vi "initialiseFields.vi"(8 "error in (no error)":errorcluster, 11 "ScanCreator in":refnum<class "ScanCreator.lvclass">) -> (0 "error out":errorcluster, 3 "ScanCreator out":refnum<class "ScanCreator.lvclass">)   [LabVIEW 2011, in "Views.lvlib" / "ScriptEditor.lvlib" / "ScanCreator.lvclass"]
uses:
  ScanCreator.lvclass
  ScanCreator.lvclass/ScanCreator.ctl
  Tools/Scripting/ScriptingEvent/ScriptEvent.lvclass
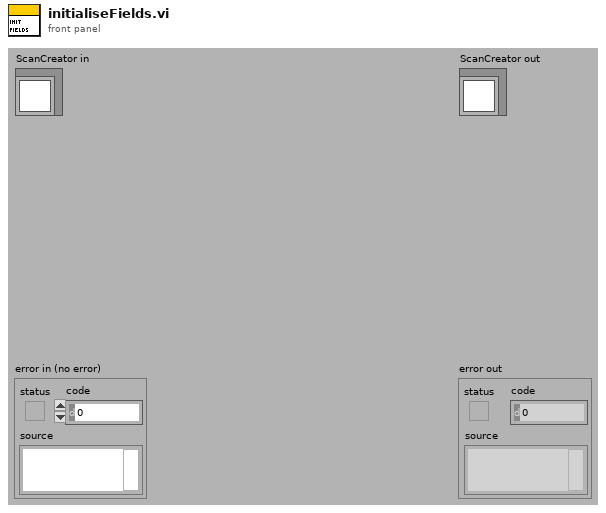
[diagram p1: front panel]
types:
  T1 = enum16{"changeValue", "pulse", "clock", "rampUp", "rampDown", "singleTone", "singleToneRamp", "playFile", "rf", "rfRamp", "delay"}
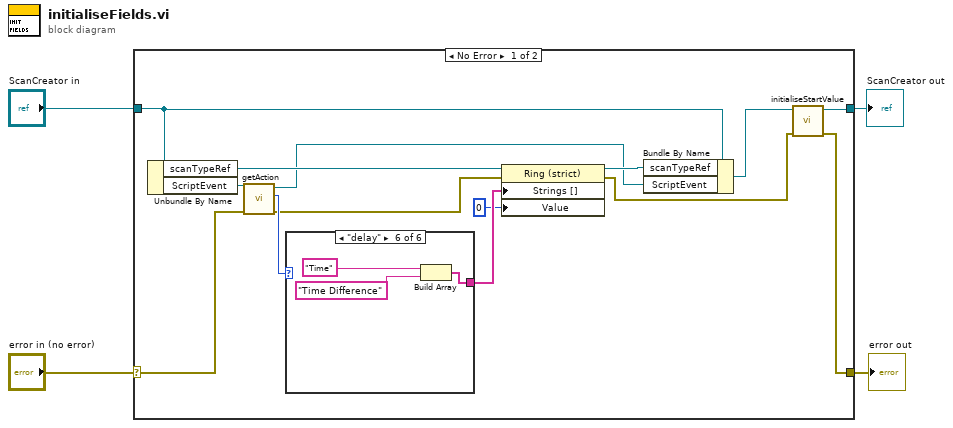
[diagram p0: block diagram]
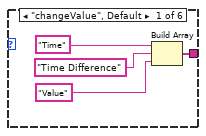
[diagram p2: hidden frame]
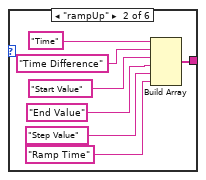
[diagram p3: hidden frame]
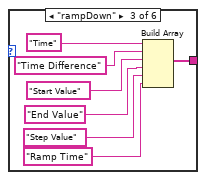
[diagram p4: hidden frame]
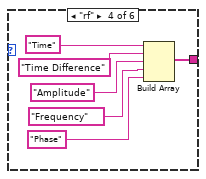
[diagram p5: hidden frame]
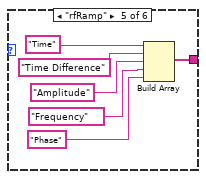
[diagram p6: hidden frame]
diagram:
  n1 = case shown="No Error" "error in (no error)" {
    selector: "error in (no error)" -> [w17 w53]
    tunnel: [w11 w53] -> w3
    tunnel: [w12 w52] -> w1
    tunnel: "ScanCreator in" -> [w10 w52]
    frame No Error {
      n2 = Unbundle By Name(w10) -> ("scanTypeRef"=w15:refnum<vi>, "ScriptEvent"=w18:refnum<class "ScriptEvent.lvclass">)
      n3 = call "getAction.vi"("error in (no error)"=w17, "ScriptEvent.lvclass in"=w18) -> ("error out"=w13:errorcluster, "action"=w16:T1, "ScriptEvent.lvclass out"=w8:refnum<class "ScriptEvent.lvclass">)  [unwired: 7 in]
      n4 = case shown="\"delay\"" w16 {
        tunnel: [w19 w28 w31 w37 w43 w49] -> w14
        frame "changeValue", Default {
          n5 = Build Array("Time", "Time Difference", "Value") -> (w19:string[])
        }
        frame "rampUp" {
          n6 = Build Array("Time", "Time Difference", "Start Value", "End Value", "Step Value", "Ramp Time") -> (w28:string[])
        }
        frame "rampDown" {
          n7 = Build Array("Time", "Time Difference", "Start Value", "End Value", "Step Value", "Ramp Time") -> (w31:string[])
        }
        frame "rf" {
          n8 = Build Array("Time", "Time Difference", "Amplitude", "Frequency", "Phase") -> (w37:string[])
        }
        frame "rfRamp" {
          n9 = Build Array("Time", "Time Difference", "Amplitude", "Frequency", "Phase") -> (w43:string[])
        }
        frame "delay" {
          n10 = Build Array("Time", "Time Difference") -> (w49:string[])
        }
      }
      n11 = property class="Ring (strict)"(reference=w15, error in=w13, "Strings []"=w14, "Value"=0) -> (reference out=w9:refnum<vi>, error out=w7:errorcluster)
      n12 = Bundle By Name(cluster=w10, "scanTypeRef"=w9, "ScriptEvent"=w8) -> (w6:refnum<class "ScanCreator.lvclass">)
      n13 = call "initialiseStartValue.vi"("error in (no error)"=w7, "ScanCreator in"=w6) -> ("error out"=w11:errorcluster, "ScanCreator out"=w12:refnum<class "ScanCreator.lvclass">)  [unwired: 8 in]
    }
    frame Error {
    }
  }
  "error out" <- w3
  "ScanCreator out" <- w1
